vi "StreamTransmitTCS.vi"() -> ()   [LabVIEW 2018]
uses:
  <vilib>/Instr/_visa.llb/VISA Configure Serial Port (Instr).vi
panel:
  out "VISA resource name out":refnum<visa-resource-name>
  in  "Input Cluster":T1={"baud rate (9600)"=2400, "VISA resource name"=""}
  out "error out 2":errorcluster
  in  "stop":bool
  out "error out":errorcluster
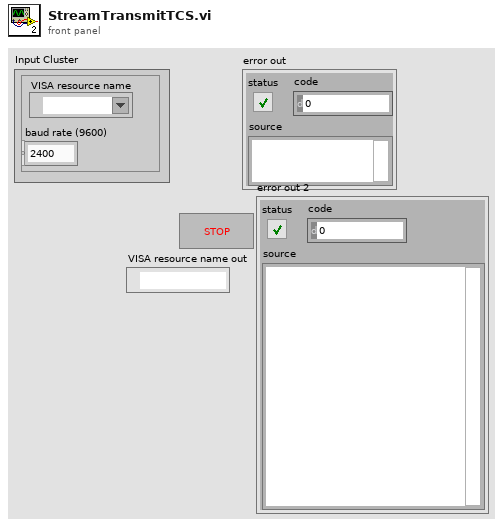
[diagram p1: front panel]
types:
  T1 = cluster{"baud rate (9600)":u32, "VISA resource name":refnum<visa-resource-name>}
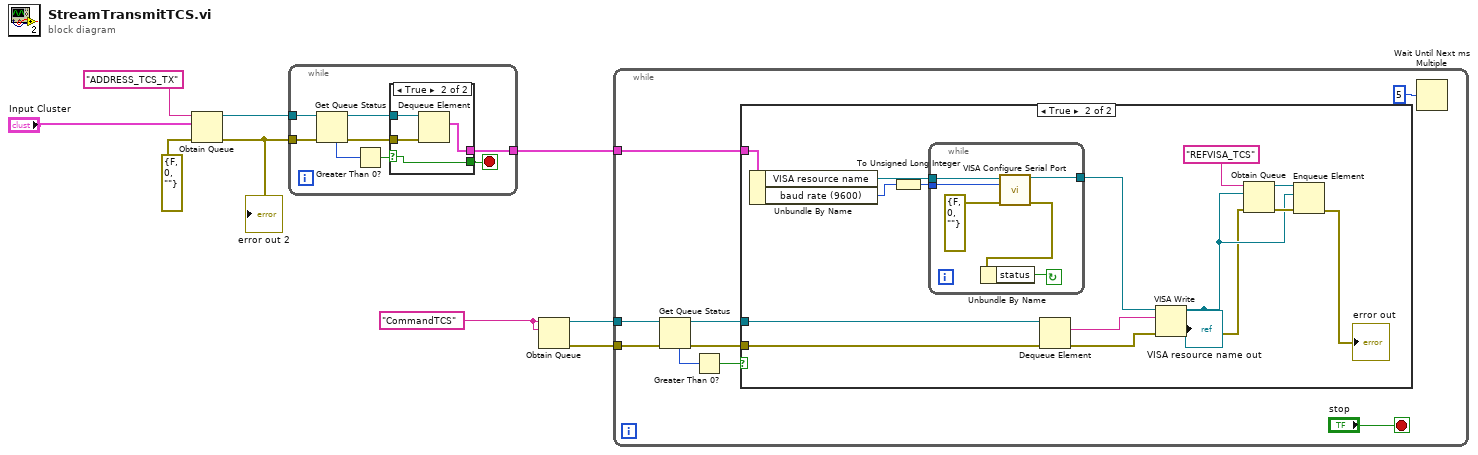
[diagram p0: block diagram]
diagram:
  w8 = "CommandTCS"
  n1 = Obtain Queue(name (unnamed)="ADDRESS_TCS_TX", element data type="Input Cluster", error in (no error)=errorcluster {"status"=FALSE, "code"=0, "source"=""}) -> (queue out=w5:refnum<queue>, error out=w6:errorcluster)  [unwired: 2 in, 1 out]
  "error out 2" <- w6
  n2 = while {
    tunnel: [w17] -> w4
    tunnel: w6 -> [w15]
    tunnel: w5 -> [w14]
    stop <- w10 stop-if-true
    n3 = Get Queue Status(queue=w14, error in (no error)=w15) -> (queue out=w13:refnum<queue>, error out=w16:errorcluster, # elements in queue=w12:i32)  [unwired: 1 in, 5 out]
    n4 = Greater Than 0?(x=w12) -> (x > 0?=w11:bool)
    n5 = case shown="True" w11 {
      selector: w11 -> [w18 w19]
      tunnel: [_ w22] -> w17
      tunnel: w16 -> [_ w21]
      tunnel: w13 -> [_ w20]
      tunnel: [w18 w19] -> w10
      frame False {
      }
      frame True {
        n6 = Dequeue Element(queue=w20, error in (no error)=w21) -> (element=w22:T1)  [unwired: 1 in, 3 out]
      }
    }
  }
  n7 = Obtain Queue(name (unnamed)=w8, element data type=w8) -> (queue out=w9:refnum<queue>, error out=w3:errorcluster)  [unwired: 3 in, 1 out]
  n8 = while {
    tunnel: w9 -> [w30]
    tunnel: w4 -> [w23]
    tunnel: w3 -> [w25]
    stop <- "stop" stop-if-true
    n9 = Get Queue Status(queue=w30, error in (no error)=w25) -> (queue out=w27:refnum<queue>, error out=w24:errorcluster, # elements in queue=w29:i32)  [unwired: 1 in, 5 out]
    n10 = Greater Than 0?(x=w29) -> (x > 0?=w28:bool)
    n11 = case shown="True" w28 {
      tunnel: w27 -> [_ w46]
      tunnel: w24 -> [_ w38]
      tunnel: w23 -> [_ w32]
      frame False {
      }
      frame True {
        n12 = Unbundle By Name(w32) -> ("VISA resource name"=w35:refnum<visa-resource-name>, "baud rate (9600)"=w36:u32)
        n13 = To Unsigned Long Integer(number=w36) -> (unsigned 32bit integer=w34:u32)
        n14 = while {
          tunnel: w34 -> [w50]
          tunnel: w35 -> [w51]
          tunnel: [w47] -> w33
          stop <- w52 continue-if-true
          n15 = call-poly "VISA Configure Serial Port"("VISA resource name"=w51, "baud rate (9600)"=w50, "error in (no error)"=errorcluster {"status"=FALSE, "code"=0, "source"=""}) -> ("VISA resource name out"=w47:refnum<visa-resource-name>, "error out"=w48:errorcluster)  [unwired: 11 in]
          n16 = Unbundle By Name(w48) -> ("status"=w52:bool)
        }
        n17 = Dequeue Element(queue=w46, error in (no error)=w38) -> (element=w41:string, error out=w37:errorcluster)  [unwired: 1 in, 2 out]
        n18 = VISA Write(VISA resource name=w33, write buffer=w41, error in (no error)=w37) -> (VISA resource name out=w40:refnum<visa-resource-name>, error out=w39:errorcluster)  [unwired: 1 out]
        "VISA resource name out" <- w40
        n19 = Obtain Queue(name (unnamed)="REFVISA_TCS", element data type=w40, error in (no error)=w39) -> (queue out=w43:refnum<queue>, error out=w44:errorcluster)  [unwired: 2 in, 1 out]
        n20 = Enqueue Element(queue=w43, element=w40, error in (no error)=w44) -> (error out=→"error out":errorcluster)  [unwired: 1 in, 2 out]
      }
    }
    n21 = Wait Until Next ms Multiple(millisecond multiple=u32 5) -> ()  [unwired: 1 out]
  }
